vi "TX Top.vi"() -> ()   [LabVIEW 2018]
uses:
  <vilib>/addons/Modulation/Analog/support/mod_Set Error Source.vi
  <vilib>/addons/Modulation/Digital/Support/Common/Validators/mod_Generate Filter Coefficients Validate.vi
  <vilib>/addons/Modulation/Digital/General/subVIs/mod_Generate Filter Coefficients.vi
  <vilib>/addons/Modulation/niDMT.lvlib
panel:
  out "Data SCs Equal within Margin?":bool[](array[boolean])
  out "Subcarriers Received":i32
  out "output bit stream, MT Modulate":i32[](array[numeric]) caption="output bit stream"
  out "size(s) 2":i32
  out "Constellation Graph":T1(graph)
  out "Waveform Chart":waveform(dbl)(graph)
  out "sampling info":cluster{"Fs":dbl, "#s":dbl}={"Fs"=1000.0, "#s"=1000.0} {"Fs" format="%.2p"}
  in  "QAM Complexity":T2(ring)
  in  "QAM Comparison":enum16{"MT Modulate", "Homebrew"}(ring)
  in  "Number of Symbols":i32=1
  in  "Samples/Symbol":i32=12
  in  "Symbol Rate":i32=1
  # "NOTE: MT Modulate misses one subcarrier for (?) reasons"
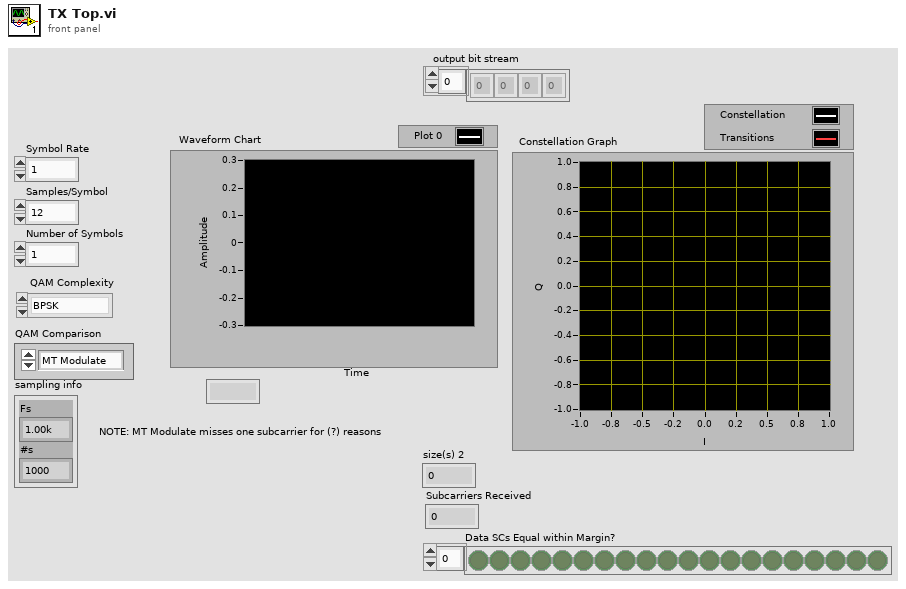
[diagram p1: front panel]
types:
  T1 = cluster{"Decimated Array":dbl[], "Decimated Array":dbl[]}[]
  T2 = enum16{"BPSK", "QPSK", "16-QAM", "64-QAM", "256-QAM"}
  T3 = enum16{"FSK", "PSK", "QAM", "MSK", "PAM", "ASK", "CPM"}
  T4 = typedef "niAMT.lvlib/Complex Data Waveform.ctl" = cluster{"t0":dbl, "dt":dbl, "Y":cdb[]}
  T5 = cluster{"constellation":dbl[], "oversampled data":dbl[]}[]
  T6 = cluster{"Samples/Symbol":i32, "symbol map":cdb[]}
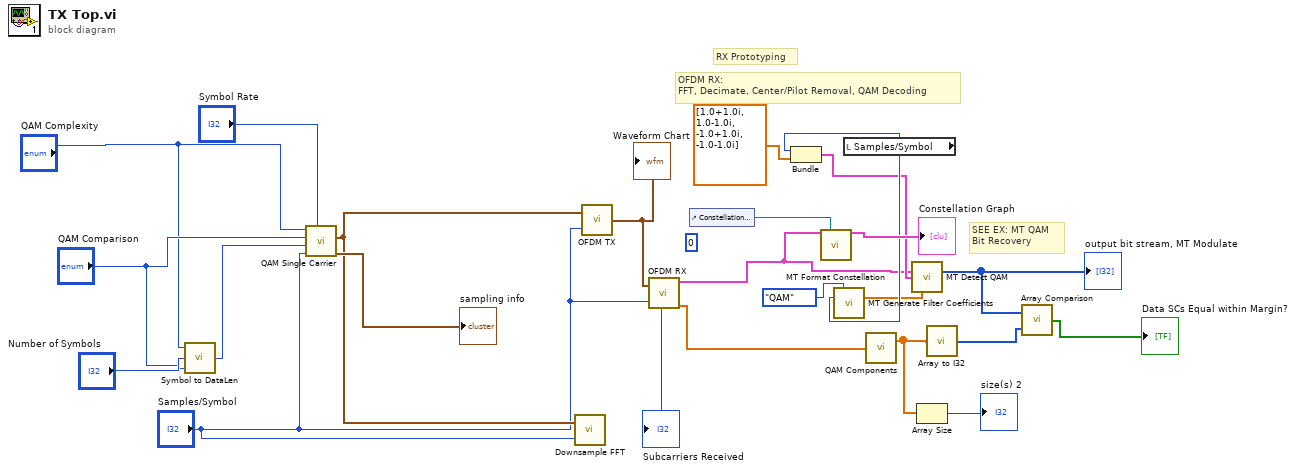
[diagram p0: block diagram]
diagram:
  (unwired) 0
  # "SEE EX: MT QAM \nBit Recovery"
  # "OFDM RX:\nFFT, Decimate, Center/Pilot Removal, QAM Decoding"
  # "RX Prototyping"
  n1 = call "Symbol to DataLen.vi"("QAM Comparison"="QAM Comparison", "Number of Symbols"="Number of Symbols", "QAM Complexity"="QAM Complexity") -> ("DataLen"=w17:i32)
  n2 = call "QAM Single Carrier.vi"("Symbol Rate"="Symbol Rate", "Samples/Symbol"="Samples/Symbol", "DataLen"=w17, "QAM Comparison"="QAM Comparison", "QAM Complexity"="QAM Complexity") -> ("sampling info"=→"sampling info":cluster{"Fs":dbl, "#s":dbl}, "Waveform"=w15:waveform(cdb))  [unwired: 2 out]
  n3 = call "Downsample FFT.vi"("Samples/Symbol"="Samples/Symbol", "FFT Received"=w15) -> ()  [unwired: 1 out]
  n4 = call "OFDM TX.vi"("Samples/Symbol"="Samples/Symbol", "Waveform"=w15) -> ("TX Signal"=w9:waveform(cdb))
  "Waveform Chart" <- w9
  n5 = call "OFDM RX.vi"("Waveform"=w9, "Samples/Symbol"="Samples/Symbol") -> ("Complex Waveform"=w7:T4, "Subcarriers Received"=→"Subcarriers Received":i32, "Out  - Digital Subcarriers"=w5:cdb[])  [unwired: 1 out]
  n6 = control-ref of="Constellation Graph"() -> (w22:refnum<vi>)
  n7 = call <vilib>:"MT Format Constellation.vi"("waveform"=w7, "constellation reference"=w22) -> ("constellation graph"=→"Constellation Graph":T5)  [unwired: 3 in, 10 out]
  n8 = local read "Samples/Symbol"() -> (w12:i32)
  n9 = Bundle("Samples/Symbol"=w12, "symbol map"=cdb[] [1.0+1.0i, 1.0-1.0i, -1.0+1.0i, -1.0-1.0i]) -> (w11:T6)  [unwired: 1 in]
  n10 = call <vilib>:"MT Generate Filter Coefficients.vi"("modulation type"=T3."QAM", "pulse shaping samples per symbol (16)"=w12) -> ("matched filter coefficients"=w10:dbl[])  [unwired: 11 in, 2 out]
  n11 = call "QAM Components.vi"("FFT Downsampled"=w5) -> ("FFT , Data"=w4:cdb[])  [unwired: 1 out]
  n12 = call <vilib>:"MT Detect QAM.vi"("input complex waveform"=w7, "QAM system parameters"=w11, "matched filter coefficients"=w10) -> ("output bit stream"=w3:i8[])  [unwired: 10 in, 2 out]
  "output bit stream, MT Modulate" <- w3
  n13 = Array Size(array=w4) -> (size(s)=→"size(s) 2":i32)
  n14 = call "Array to I32.vi"("DBL Array"=w4) -> ("I32 Array"=w2:i32[])
  n15 = call "Array Comparison.vi"("Bit STream 2"=w2, "Bit Stream 1"=w3) -> ("Bit Stream Comparison"=→"Data SCs Equal within Margin?":bool[])
